vi "Module Init.vi"(8 "error in (no error)":errorcluster, 11 "ToggleTestModule in":refnum<class "ToggleTestModule.lvclass">) -> (0 "error out":errorcluster, 3 "ToggleTestModule out":refnum<class "ToggleTestModule.lvclass">)   [LabVIEW 2020, in "VolatusScratch.lvlib" / "ToggleTestModule.lvclass"]
uses:
  ToggleTestModule.lvclass
  ToggleTestModule.lvclass/ToggleTestModule.ctl
  Volatus/Module/Module.lvclass
  C:/dev/lv20CE/relink/lv-volatus/Volatus/Module/Module.lvclass
  C:/dev/lv20CE/relink/lv-volatus/VolatusScratch/ToggleTestModule/ToggleTestModule.lvclass
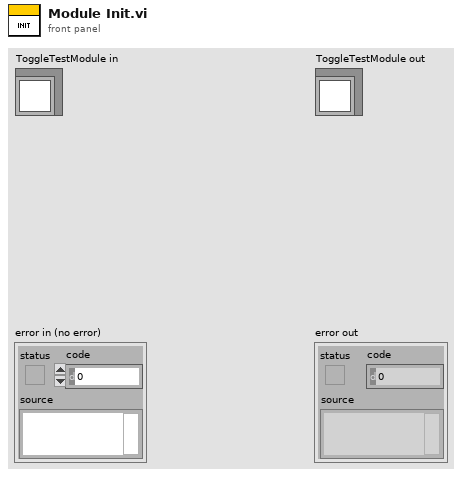
[diagram p1: front panel]
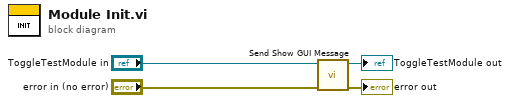
[diagram p0: block diagram]
diagram:
  n1 = call "Send Show GUI Message.vi"("error in (no error)"="error in (no error)", "Module in"="ToggleTestModule in") -> ("error out"=→"error out":errorcluster, "Module out"=→"ToggleTestModule out":refnum<class "ToggleTestModule.lvclass">)  [unwired: 8 in]
